vi "FPGA Selection.vi"() -> ()   [LabVIEW 2020]
uses:
  Globals/FPGA Globals.vi
panel:
  in  "Confirm":bool
  in  "Controller MAC Address":string
  out "PC MAC Address":string
  in  "Select PC Adapter MAC Address":u16(ring)
  out "Ports Detected by PCAP":string[](array[string])
  out "PC Ethernet Port No. (PCAP count)":i32
  out "FPGA MAC":string
  out "System Clock(MHz)":dbl
  in  "Select Ethernet Port (winPCAP)":u16(ring)
  out "Shell Output":string
  out "Port MAC Addresses":string[](array[string])
  # "PLEASE SELECT AND CONFIRM BEFORE GOING BACK TO THE MAIN SCREEN"
  # "Available"
  # "Available"
  # "Settings to use"
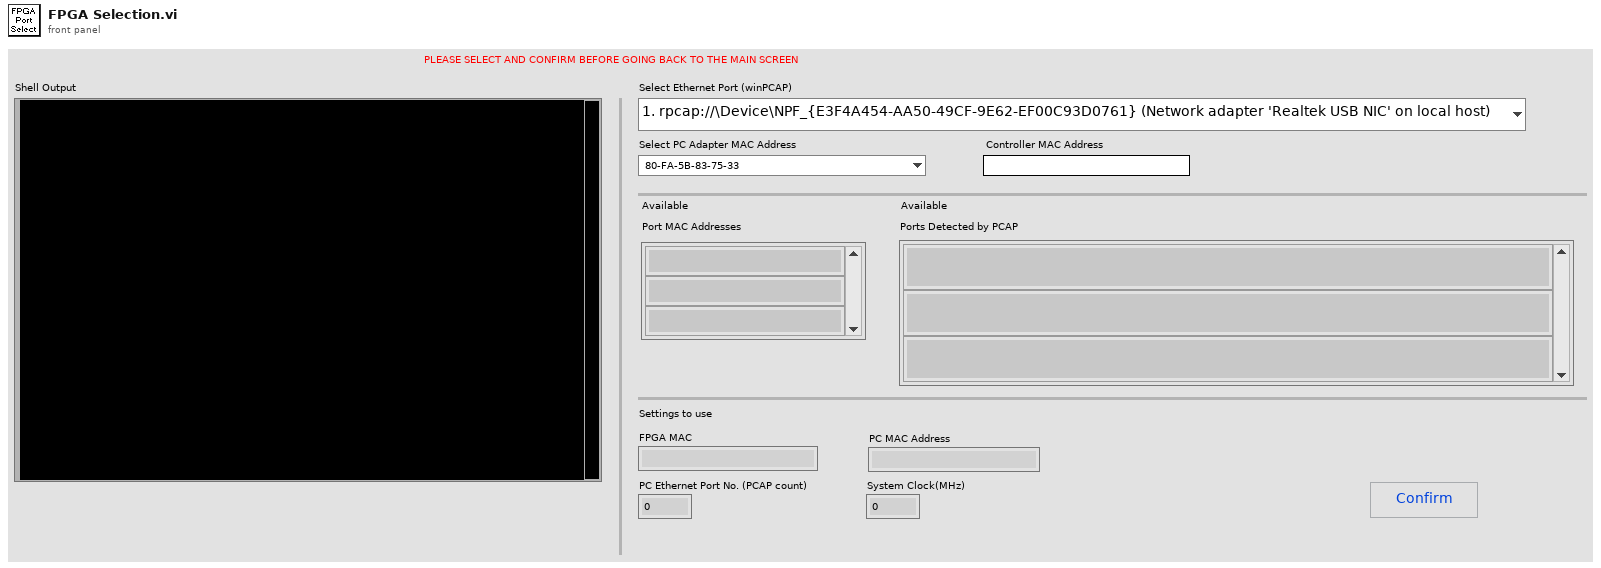
[diagram p1: front panel]
types:
  T1 = typedef "FPGA Settings.ctl" = cluster{"System Clock(MHz)":dbl, "FPGA MAC 1":string, "Port Number 1":i32, "Port Number 2":i32, "FPGA MAC 2":string, "PC MAC Address":string}
  T2 = typedef "FPGA_DAQ_settings.ctl" = cluster{"Use FlexRIO Trigger":bool, "RIO Resource Name":string, "Use detected RIO resource":bool, "Ethernet Card WinPCap Port ":i16, "Adapter Module":T3, "FPGA Card":T4}
  T3 = typedef "FPGA_adapter_type.ctl" = enum16{"5772-DC", "5772-AC"}
  T4 = typedef "FPGA_card_type.ctl" = enum16{"7976R", "7975R", "7966R"}
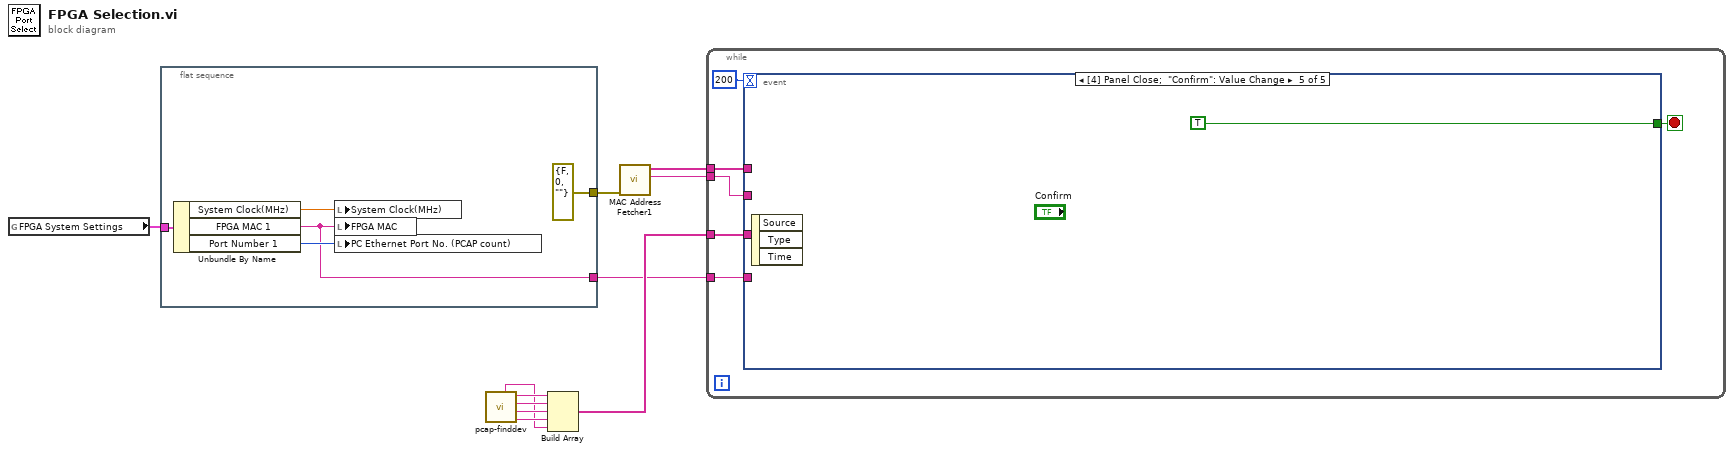
[diagram p0: block diagram]
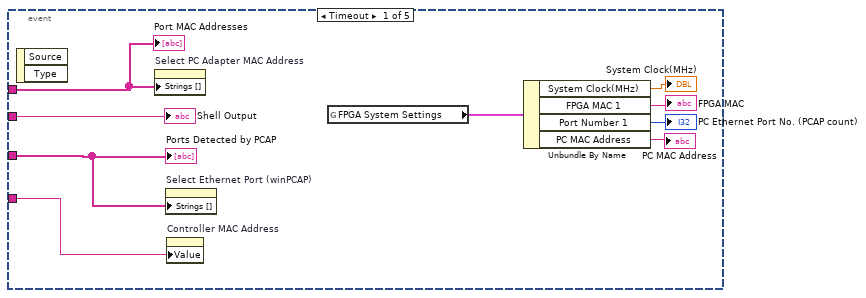
[diagram p2: hidden frame]
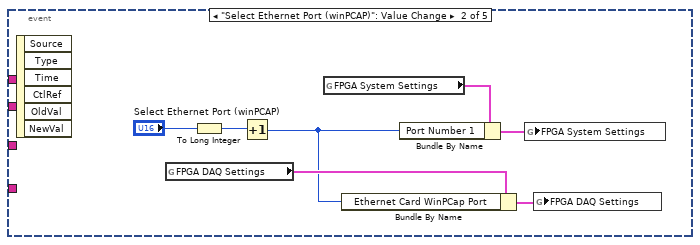
[diagram p3: hidden frame]
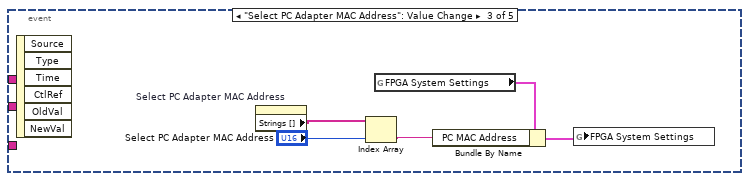
[diagram p4: hidden frame]
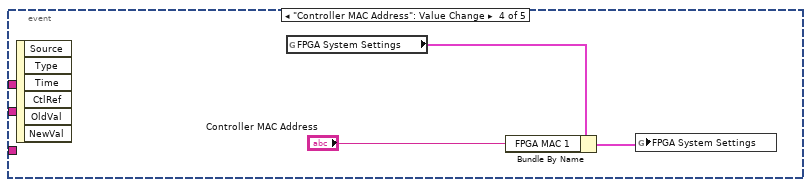
[diagram p5: hidden frame]
diagram:
  n1 = global read "FPGA Globals.vi" "FPGA System Settings"() -> (w9:T1)
  n2 = flat-sequence {
    tunnel: w9 -> [w16]
    tunnel: [errorcluster {"status"=FALSE, "code"=0, "source"=""} ("error in (no error)")] -> w2
    tunnel: [w12] -> w1
    frame #0 {
      n3 = Unbundle By Name(w16) -> ("System Clock(MHz)"=w15:dbl, "FPGA MAC 1"=w12:string, "Port Number 1"=w14:i32)
      n4 = local write "System Clock(MHz)"(w15) -> ()
      n5 = local write "FPGA MAC"(w12) -> ()
      n6 = local write "PC Ethernet Port No. (PCAP count)"(w14) -> ()
    }
  }
  n7 = call "pcap-finddev.vi"() -> ("String 4"=w5:string, "String 3"=w6:string, "String 2"=w7:string, "String"=w8:string, "String 5"=w3:string)  [unwired: 1 in]
  n8 = Build Array(w8, w7, w6, w5, w3) -> (w4:string[])
  n9 = call "MAC Address Fetcher1.vi"("error in (no error)"=w2) -> ("Shell Output"=w10:string, "MAC Addresses"=w11:string[])  [unwired: 8 in, 1 out]
  n10 = while {
    tunnel: w11 -> [w19]
    tunnel: w10 -> [w20]
    tunnel: w4 -> [w18]
    tunnel: w1 -> [w17]
    stop <- w21 stop-if-true
    n11 = event shown="[4] Panel Close;  \"Confirm\": Value Change" {
      selector: _ -> [_ _ _ _ _]
      dyn-events: _ -> [_ _ _ _ _]
      timeout: 200 -> [_ _ _ _ _]
      tunnel: [_ _ _ _ TRUE] -> w21
      tunnel: w20 -> [w31 _ _ _ _]
      tunnel: w19 -> [w29 _ _ _ _]
      tunnel: w18 -> [w30 _ _ _ _]
      tunnel: w17 -> [w23 _ _ _ _]
      event Timeout {
        n12 = event-data() -> ()  [unwired: 1 in, 2 out]
        n13 = property on="Select PC Adapter MAC Address" class="Ring (strict)"("Strings []"=w29) -> ()  [unwired: 2 in, 2 out]
        n14 = property on="Select Ethernet Port (winPCAP)" class="Ring (strict)"("Strings []"=w30) -> ()  [unwired: 2 in, 2 out]
        n15 = property on="Controller MAC Address" class="Str"("Value"=w23) -> ()  [unwired: 2 in, 2 out]
        n16 = global read "FPGA Globals.vi" "FPGA System Settings"() -> (w24:T1)
        n17 = Unbundle By Name(w24) -> ("System Clock(MHz)"=→"System Clock(MHz)":dbl, "FPGA MAC 1"=→"FPGA MAC":string, "Port Number 1"=→"PC Ethernet Port No. (PCAP count)":i32, "PC MAC Address"=→"PC MAC Address":string)
        "Port MAC Addresses" <- w29
        "Shell Output" <- w31
        "Ports Detected by PCAP" <- w30
      }
      event "Select Ethernet Port (winPCAP)": Value Change {
        n18 = event-data() -> ()  [unwired: 1 in, 6 out]
        n19 = global read "FPGA Globals.vi" "FPGA DAQ Settings"() -> (w34:T2)
        n20 = To Long Integer(number="Select Ethernet Port (winPCAP)") -> (32bit integer=w38:i32)
        n21 = Increment(x=w38) -> (x+1=w33:i32)
        n22 = global read "FPGA Globals.vi" "FPGA System Settings"() -> (w35:T1)
        n23 = Bundle By Name(cluster=w34, "Ethernet Card WinPCap Port"=w33) -> (w32:T2)
        n24 = Bundle By Name(cluster=w35, "Port Number 1"=w33) -> (w36:T1)
        n25 = global write "FPGA Globals.vi" "FPGA System Settings"(w36) -> ()
        n26 = global write "FPGA Globals.vi" "FPGA DAQ Settings"(w32) -> ()
      }
      event "Select PC Adapter MAC Address": Value Change {
        n27 = event-data() -> ()  [unwired: 1 in, 6 out]
        n28 = property on="Select PC Adapter MAC Address" class="Ring (strict)"() -> ("Strings []"=w39:string[])  [unwired: 2 in, 2 out]
        n29 = Index Array(array=w39, index="Select PC Adapter MAC Address") -> (element=w41:string)
        n30 = global read "FPGA Globals.vi" "FPGA System Settings"() -> (w42:T1)
        n31 = Bundle By Name(cluster=w42, "PC MAC Address"=w41) -> (w40:T1)
        n32 = global write "FPGA Globals.vi" "FPGA System Settings"(w40) -> ()
      }
      event "Controller MAC Address": Value Change {
        n33 = event-data() -> ()  [unwired: 1 in, 6 out]
        n34 = global read "FPGA Globals.vi" "FPGA System Settings"() -> (w46:T1)
        n35 = Bundle By Name(cluster=w46, "FPGA MAC 1"="Controller MAC Address") -> (w45:T1)
        n36 = global write "FPGA Globals.vi" "FPGA System Settings"(w45) -> ()
      }
      event Panel Close; "Confirm": Value Change {
        n37 = event-data() -> ()  [unwired: 1 in, 3 out]
      }
    }
  }
